vi "ATM_FP.Comminication_Command_RW.vi"(0 "VISA":refnum<visa-resource-name>, 1 "openPort?":bool=TRUE, 5 "Command":T1, 9 "fpID(StoreChar,Delete)":u16, 11 "error in (no error)":errorcluster) -> (2 "CorrectFormat":bool, 3 "returnParameter":string, 4 "VISA(Duplicate)":refnum<visa-resource-name>, 6 "read buffer":string, 8 "reponseOK?":bool, 10 "confirmationMsg":string, 15 "error IO":errorcluster)   [LabVIEW 2020]
uses:
  __ATM__FP__COMMUNICATION__COMMAND__.ctl
  <vilib>/Instr/_visa.llb/VISA Configure Serial Port (Instr).vi
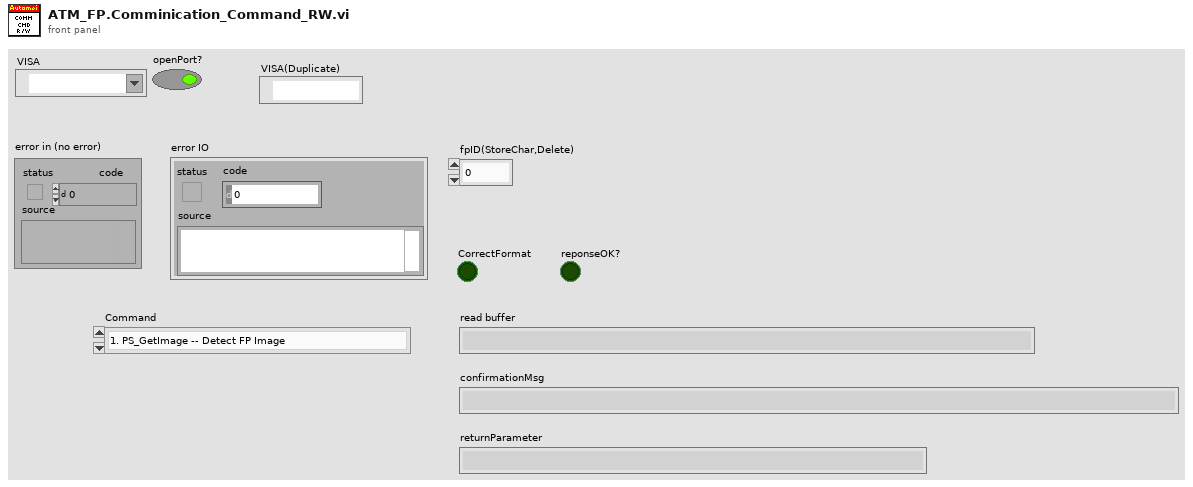
[diagram p1: front panel]
types:
  T1 = typedef "__ATM__FP__COMMUNICATION__COMMAND__.ctl" = enum16{"1. PS_GetImage -- Detect FP Image", "2. PS_GenChar -- Generate FP Template from Image [BufferChar1]", "2. PS_GenChar -- Generate FP Template from Image [BufferChar2]", "3. PS_Match -- Compare 2 FP Template", "4. PS_Search -- Search fingerprint", "5. PS_RegModel -- Generate template", "6. PS_StoreChar -- Store template", "7. PS_LoadChar -- FP Database -->Feature Buffer", "8. PS_UpChar --  Upload Feature Buff --> PC", "12. PS_DeletChar -- Delete template", "13. PS_Empty -- Delete all FP templates", "15. S_ReadSysPara -- Read system basic parameters"}
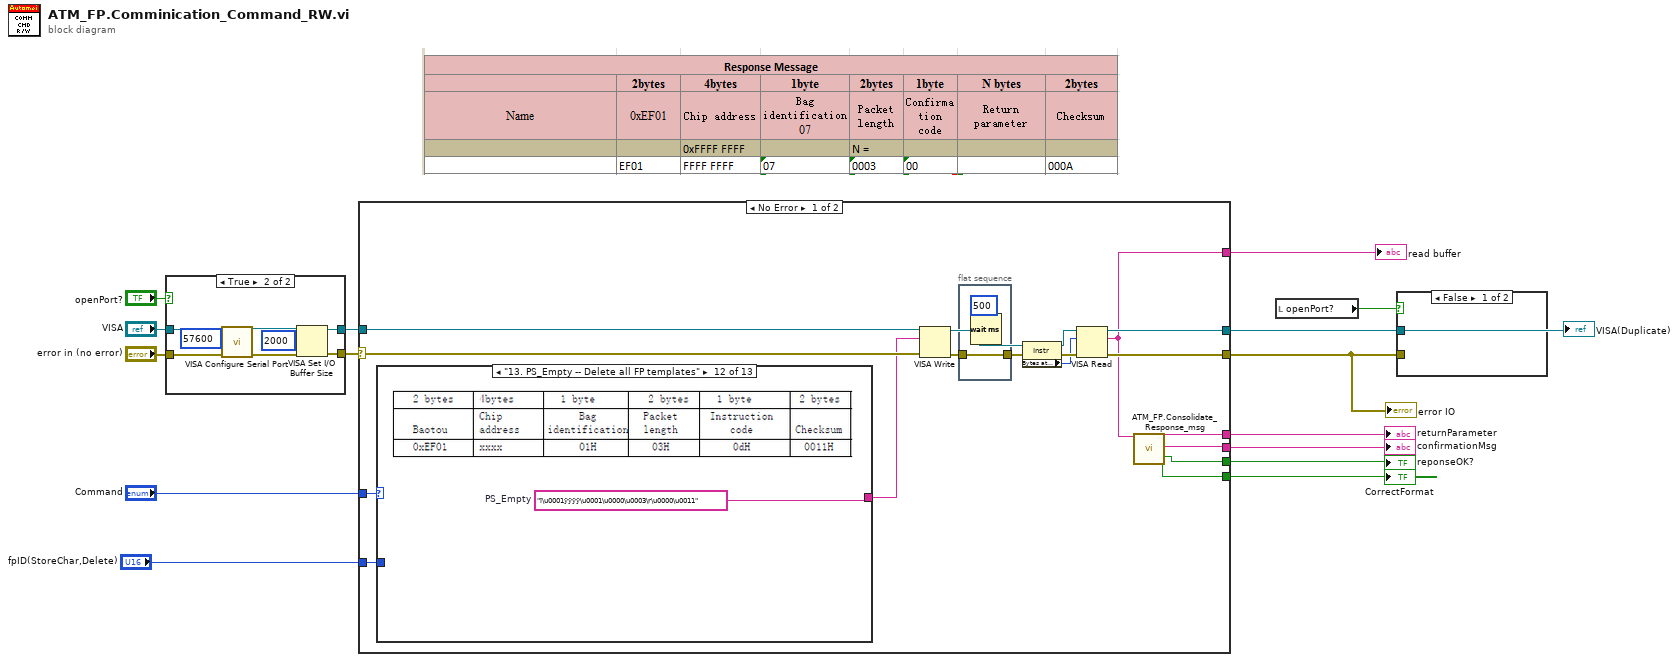
[diagram p0: block diagram]
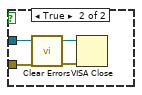
[diagram p2: hidden frame]
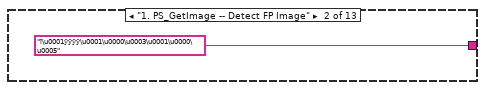
[diagram p5: hidden frame]
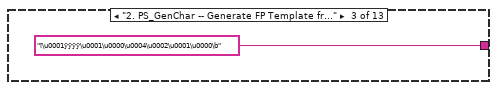
[diagram p6: hidden frame]
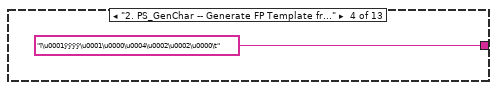
[diagram p7: hidden frame]
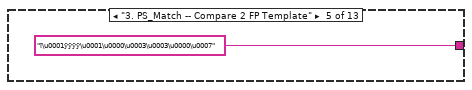
[diagram p8: hidden frame]
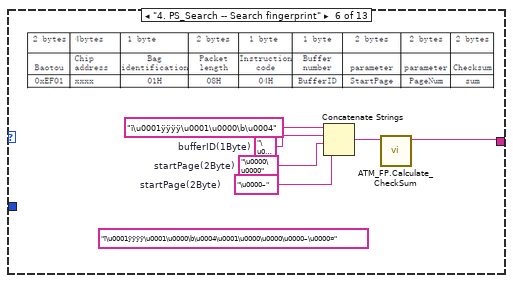
[diagram p9: hidden frame]
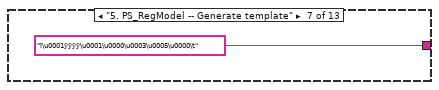
[diagram p10: hidden frame]
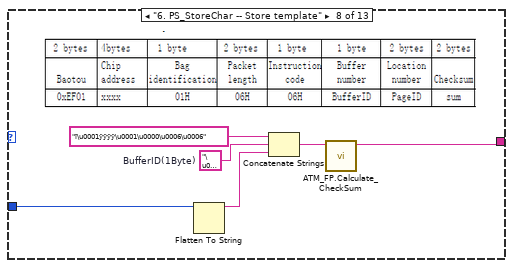
[diagram p11: hidden frame]
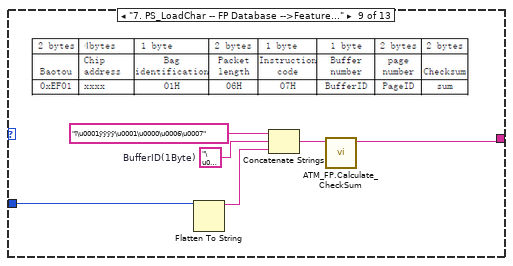
[diagram p12: hidden frame]
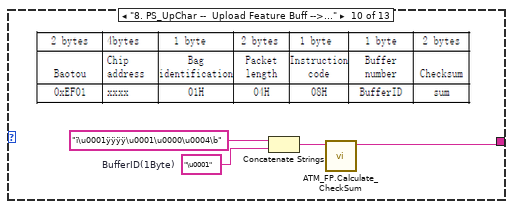
[diagram p13: hidden frame]
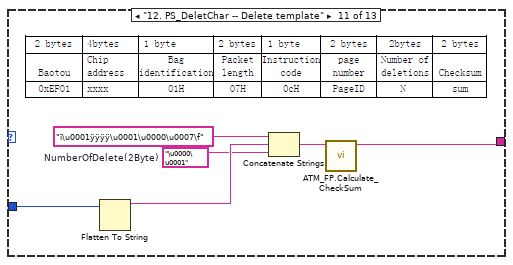
[diagram p14: hidden frame]
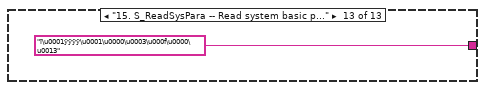
[diagram p15: hidden frame]
diagram:
  n1 = case shown="True" "openPort?" {
    tunnel: "VISA" -> [w17 w24]
    tunnel: "error in (no error)" -> [w16 w23]
    tunnel: [w17 w20] -> w11
    tunnel: [w16 w18] -> w10
    frame False {
    }
    frame True {
      n2 = call-poly "VISA Configure Serial Port"("VISA resource name"=w24, "baud rate (9600)"=u32 57600, "error in (no error)"=w23) -> ("VISA resource name out"=w21:refnum<visa-resource-name>, "error out"=w19:errorcluster)  [unwired: 11 in]
      n3 = VISA Set I/O Buffer Size(VISA resource name=w21, size (4096)=u32 2000 ("大小(4096)"), error in (no error)=w19) -> (VISA resource name out=w20:refnum<visa-resource-name>, error out=w18:errorcluster)  [unwired: 1 in]
    }
  }
  n4 = case shown="No Error" w10 {
    selector: w10 -> [w40 w82]
    tunnel: [w43 w82] -> w12
    tunnel: [w42 w81] -> w15
    tunnel: w11 -> [w41 w81]
    tunnel: "Command" -> [w38 _]
    tunnel: [w29 _] -> w8
    tunnel: [w31 _] -> w7
    tunnel: [w30 _] -> w6
    tunnel: [w28 _] -> w5
    tunnel: [w27 _] -> w4
    tunnel: "fpID(StoreChar,Delete)" -> [w26 _]
    frame No Error {
      n5 = case shown="\"13. PS_Empty -- Delete all FP templates\"" w38 {
        tunnel: [_ "ï\u0001ÿÿÿÿ\u0001\u0000\u0003\u0001\u0000\u0005" "ï\u0001ÿÿÿÿ\u0001\u0000\u0004\u0002\u0001\u0000\b" "ï\u0001ÿÿÿÿ\u0001\u0000\u0004\u0002\u0002\u0000\t" "ï\u0001ÿÿÿÿ\u0001\u0000\u0003\u0003\u0000\u0007" w48 "ï\u0001ÿÿÿÿ\u0001\u0000\u0003\u0005\u0000\t" w58 w64 w68 w74 w77 "ï\u0001ÿÿÿÿ\u0001\u0000\u0003\u000f\u0000\u0013"] -> w37
        tunnel: w26 -> [_ _ _ _ _ _ _ w55 w61 _ w73 _ _]
        frame Default {
        }
        frame "1. PS_GetImage -- Detect FP Image" {
        }
        frame "2. PS_GenChar -- Generate FP Template from Image [BufferChar1]" {
        }
        frame "2. PS_GenChar -- Generate FP Template from Image [BufferChar2]" {
        }
        frame "3. PS_Match -- Compare 2 FP Template" {
        }
        frame "4. PS_Search -- Search fingerprint" {
          w49 = "\u0000–"  # startPage(2Byte)
          w50 = "\u0000\u0000"  # startPage(2Byte)
          w51 = "\u0001"  # bufferID(1Byte)
          (unwired) "ï\u0001ÿÿÿÿ\u0001\u0000\b\u0004\u0001\u0000\u0000\u0000–\u0000¤"
          n6 = Concatenate Strings("ï\u0001ÿÿÿÿ\u0001\u0000\b\u0004", w51, w50, w49) -> (w52:string)
          n7 = call "ATM_FP.Calculate_CheckSum.vi"("DataPacket"=w52) -> ("DataPacket+Checksum"=w48:string)  [unwired: 9 in, 1 out]
        }
        frame "5. PS_RegModel -- Generate template" {
        }
        frame "6. PS_StoreChar -- Store template" {
          w57 = "\u0001"  # BufferID(1Byte)
          n8 = Flatten To String(anything=w55) -> (data string=w56:string)  [unwired: 3 in, 2 out]
          n9 = Concatenate Strings("ï\u0001ÿÿÿÿ\u0001\u0000\u0006\u0006", w57, w56) -> (w59:string)
          n10 = call "ATM_FP.Calculate_CheckSum.vi"("DataPacket"=w59) -> ("DataPacket+Checksum"=w58:string)  [unwired: 9 in, 1 out]
        }
        frame "7. PS_LoadChar -- FP Database -->Feature Buffer" {
          w63 = "\u0001"  # BufferID(1Byte)
          n11 = Flatten To String(anything=w61) -> (data string=w62:string)  [unwired: 3 in, 2 out]
          n12 = Concatenate Strings("ï\u0001ÿÿÿÿ\u0001\u0000\u0006\u0007", w63, w62) -> (w65:string)
          n13 = call "ATM_FP.Calculate_CheckSum.vi"("DataPacket"=w65) -> ("DataPacket+Checksum"=w64:string)  [unwired: 9 in, 1 out]
        }
        frame "8. PS_UpChar --  Upload Feature Buff --> PC" {
          w67 = "\u0001"  # BufferID(1Byte)
          n14 = Concatenate Strings("ï\u0001ÿÿÿÿ\u0001\u0000\u0004\b", w67) -> (w69:string)
          n15 = call "ATM_FP.Calculate_CheckSum.vi"("DataPacket"=w69) -> ("DataPacket+Checksum"=w68:string)  [unwired: 9 in, 1 out]
        }
        frame "12. PS_DeletChar -- Delete template" {
          w71 = "\u0000\u0001"  # NumberOfDelete(2Byte)
          n16 = Flatten To String(anything=w73) -> (data string=w72:string)  [unwired: 3 in, 2 out]
          n17 = Concatenate Strings("ï\u0001ÿÿÿÿ\u0001\u0000\u0007\f", w72, w71) -> (w75:string)
          n18 = call "ATM_FP.Calculate_CheckSum.vi"("DataPacket"=w75) -> ("DataPacket+Checksum"=w74:string)  [unwired: 9 in, 1 out]
        }
        frame "13. PS_Empty -- Delete all FP templates" {
          w77 = "ï\u0001ÿÿÿÿ\u0001\u0000\u0003\r\u0000\u0011"  # PS_Empty
        }
        frame "15. S_ReadSysPara -- Read system basic parameters" {
        }
      }
      n19 = VISA Write(VISA resource name=w41, write buffer=w37, error in (no error)=w40) -> (VISA resource name out=w34:refnum<visa-resource-name>, error out=w39:errorcluster)  [unwired: 1 out]
      n20 = flat-sequence {
        tunnel: w39 -> [w80]
        tunnel: [w80] -> w35
        frame #0 {
          n21 = Wait (ms)(milliseconds to wait=u32 500) -> ()  [unwired: 1 out]
        }
      }
      n22 = property class="Instr"(reference=w34, error in=w35) -> (reference out=w33:refnum<visa-resource-name>, error out=w36:errorcluster, "Bytes at Port"=w32:u32)
      n23 = VISA Read(VISA resource name=w33, byte count=w32, error in (no error)=w36) -> (VISA resource name out=w42:refnum<visa-resource-name>, read buffer=w27:string, error out=w43:errorcluster)  [unwired: 1 out]
      n24 = call "ATM_FP.Consolidate_Response_msg.vi"("ResponseMessage"=w27) -> ("returnParameter"=w28:string, "confirmationMsg"=w31:string, "responseOK?"=w30:bool, "Match"=w29:bool)  [unwired: 13 in, 2 out]
    }
    frame Error {
    }
  }
  "error IO" <- w12
  "CorrectFormat" <- w8
  "confirmationMsg" <- w7
  "reponseOK?" <- w6
  "returnParameter" <- w5
  "read buffer" <- w4
  "VISA(Duplicate)" <- w15
  n25 = local read "openPort?"() -> (w2:bool)
  n26 = case shown="False" w2 {
    tunnel: w15 -> [_ w85]
    tunnel: w12 -> [_ w84]
    frame False {
    }
    frame True {
      n27 = call <vilib>:"Clear Errors.vi"("error in (no error)"=w84) -> ("error out"=w83:errorcluster)  [unwired: 5 in, 1 out]
      n28 = VISA Close(VISA resource name=w85, error in (no error)=w83) -> ()  [unwired: 1 out]
    }
  }
